vi "DarkLifetime.vi"() -> ()   [LabVIEW 2009]
panel:
  out "Run Number":i32
  in  "Runs":u32
  out "Loading":bool
  out "Percentage Kept":dbl
  in  "Ion Threshold":i32
  in  "Wait Time (ms)":u32
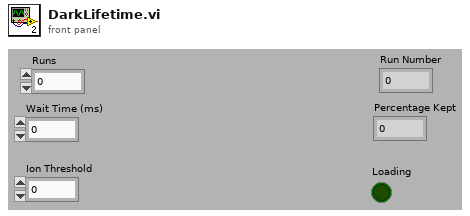
[diagram p1: front panel]
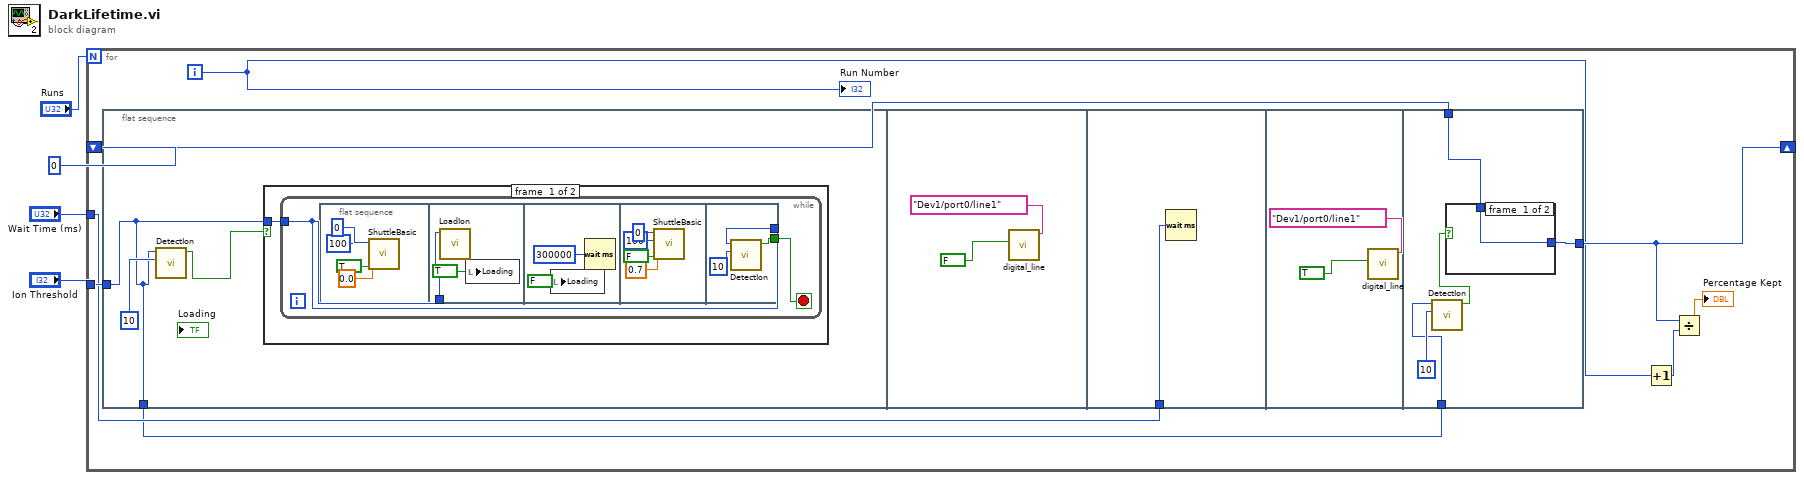
[diagram p0: block diagram]
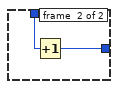
[diagram p3: hidden frame]
diagram:
  n1 = for {
    N: "Runs" -> [_]
    shift-right: [w10] -> _
    shift-left: 0 -> [w12]
    tunnel: "Wait Time (ms)" -> [w7]
    tunnel: "Ion Threshold" -> [w8]
    i -> [w6]
    n2 = flat-sequence {
      tunnel: w8 -> [w14]
      tunnel: [w14] -> w5
      tunnel: w7 -> [w36]
      tunnel: w12 -> [w43]
      tunnel: [w42] -> w10
      tunnel: w5 -> [w40]
      frame #0 {
        n3 = call "DetectIon.vi"("Samples per averaging\nblock"=10 ("Samples per averaging\nblock"), "Threshold"=w14) -> ("Ion"=w13:bool)  [unwired: 9 in]
        n4 = case shown="False" w13 {
          tunnel: w14 -> [w16 _]
          frame #0 {
            n5 = while {
              tunnel: w16 -> [w18]
              stop <- w17 stop-if-true
              n6 = flat-sequence {
                tunnel: w18 -> [w24]
                tunnel: w18 -> [w32]
                tunnel: [w31] -> w17
                frame #0 {
                  n7 = call "ShuttleBasic.vi"("Piezo Voltage"=0.0, "Reverse"=TRUE, "End"=100, "Start"=0) -> ()  [unwired: 8 in]
                }
                frame #1 {
                  n8 = call "LoadIon.vi"("Threshold"=w24) -> ()  [unwired: 10 in, 1 out]
                  n9 = local write "Loading"(TRUE ("Loading")) -> ()
                }
                frame #2 {
                  n10 = local write "Loading"(FALSE ("Loading")) -> ()
                  n11 = Wait (ms)(milliseconds to wait=u32 300000) -> ()  [unwired: 1 out]
                }
                frame #3 {
                  n12 = call "ShuttleBasic.vi"("Piezo Voltage"=0.7, "Reverse"=FALSE, "End"=100, "Start"=0) -> ()  [unwired: 8 in]
                }
                frame #4 {
                  n13 = call "DetectIon.vi"("Samples per averaging\nblock"=10 ("Samples per averaging\nblock"), "Threshold"=w32) -> ("Ion"=w31:bool)  [unwired: 9 in]
                }
              }
            }
          }
          frame #1 {
          }
        }
      }
      frame #1 {
        n14 = call "digital_line.vi"("NewVal"=FALSE, "lines"=tag "Dev1/port0/line1") -> ()  [unwired: 2 in]
      }
      frame #2 {
        n15 = Wait (ms)(milliseconds to wait=w36) -> ()  [unwired: 1 out]
      }
      frame #3 {
        n16 = call "digital_line.vi"("NewVal"=TRUE, "lines"=tag "Dev1/port0/line1") -> ()  [unwired: 2 in]
      }
      frame #4 {
        n17 = call "DetectIon.vi"("Samples per averaging\nblock"=10 ("Samples per averaging\nblock"), "Threshold"=w40) -> ("Ion"=w39:bool)  [unwired: 9 in]
        n18 = case shown="False" w39 {
          tunnel: w43 -> [w44 w46]
          tunnel: [w44 w45] -> w42
          frame #0 {
          }
          frame #1 {
            n19 = Increment(x=w46) -> (x+1=w45:i32)
          }
        }
      }
    }
    n20 = Increment(x=w6) -> (x+1=w9:i32)
    n21 = Divide(x=w10, y=w9) -> (x/y=→"Percentage Kept":dbl)
    "Run Number" <- w6
  }
